vi "decodeObject.vi"(8 "error in (no error)":errorcluster, 10 "ByteArray":u8[](array[numeric])) -> (0 "error out":errorcluster, 1 "Variant":variant, 2 "RemainingBytes":u8[](array[numeric]), 3 "Type":string)   [LabVIEW 2016, in "MsgPack.lvlib"]
uses:
  MsgPack.lvlib
  <vilib>/Utility/error.llb/Error Cluster From Error Code.vi
  <vilib>/ErrorRing/Error Ring.xnode
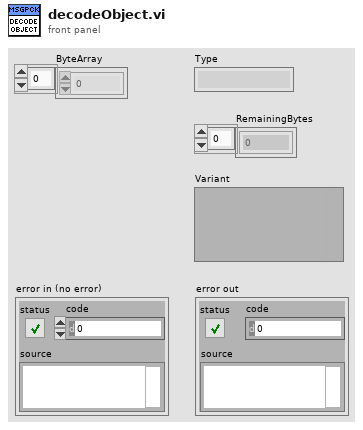
[diagram p1: front panel]
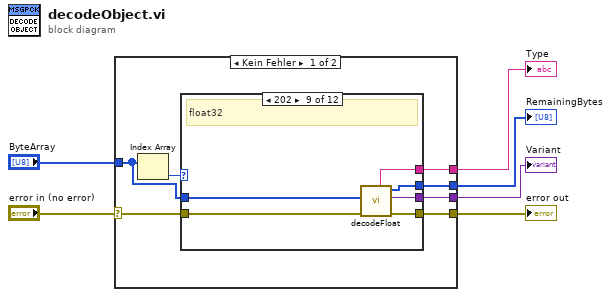
[diagram p0: block diagram]
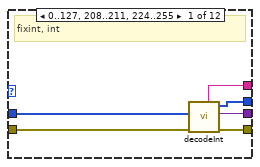
[diagram p2: hidden frame]
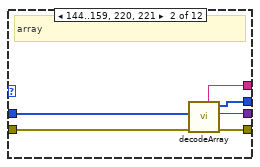
[diagram p3: hidden frame]
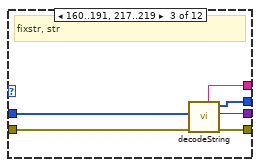
[diagram p4: hidden frame]
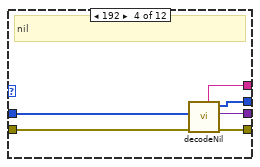
[diagram p5: hidden frame]
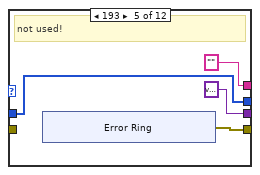
[diagram p6: hidden frame]
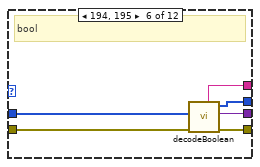
[diagram p7: hidden frame]
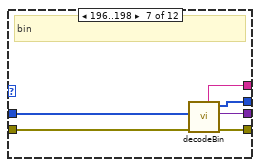
[diagram p8: hidden frame]
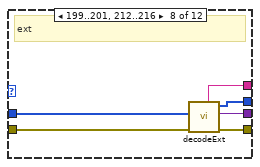
[diagram p9: hidden frame]
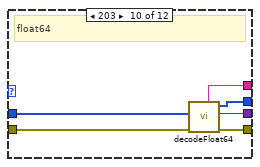
[diagram p10: hidden frame]
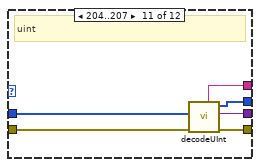
[diagram p11: hidden frame]
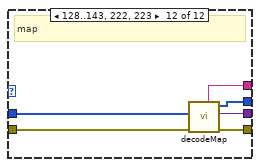
[diagram p12: hidden frame]
diagram:
  n1 = case shown="Kein Fehler" "error in (no error)" {
    selector: "error in (no error)" -> [w7 w90]
    tunnel: "ByteArray" -> [w12 w89]
    tunnel: [w11 _] -> w5
    tunnel: [w10 _] -> w4
    tunnel: [w9 w89] -> w3
    tunnel: [w8 w90] -> w2
    frame No Error {
      n2 = Index Array(array=w12) -> (element=w13:u8)  [unwired: 1 in]
      n3 = case shown="202" w13 {
        tunnel: w12 -> [w19 w24 w31 w34 w38 w52 w58 w64 w70 w76 w82 w88]
        tunnel: [w17 w22 w29 w37 w41 w50 w56 w62 w68 w74 w80 w84] -> w8
        tunnel: [w18 w21 w30 w36 variant ("variant") w51 w57 w63 w69 w75 w81 w86] -> w11
        tunnel: w7 -> [w16 w25 w26 w35 _ w49 w53 w59 w65 w71 w77 w87]
        tunnel: [w15 w23 w28 w33 w38 w47 w55 w61 w67 w72 w78 w85] -> w9
        tunnel: [w14 w20 w27 w32 "" ("Type") w48 w54 w60 w66 w73 w79 w83] -> w10
        frame 0..127, 208..211, 224..255 {
          # "fixint, int"
          n4 = call "decodeInt.vi"("error in (no error)"=w16, "ByteArray"=w19) -> ("error out"=w17:errorcluster, "variant"=w18:variant, "RemainingBytes"=w15:u8[], "Type"=w14:string)  [unwired: 5 in, 1 out]
        }
        frame 144..159, 220, 221 {
          # "array"
          n5 = call "decodeArray.vi"("error in (no error)"=w25, "ByteArray"=w24) -> ("error out"=w22:errorcluster, "variant"=w21:variant, "ByteArray"=w23:u8[], "Type"=w20:string)  [unwired: 6 in]
        }
        frame 160..191, 217..219 {
          # "fixstr, str"
          n6 = call "decodeString.vi"("error in (no error)"=w26, "ByteArray"=w31) -> ("error out"=w29:errorcluster, "variant"=w30:variant, "RemainingBytes"=w28:u8[], "Type"=w27:string)  [unwired: 5 in, 1 out]
        }
        frame 192 {
          # "nil"
          n7 = call "decodeNil.vi"("error in (no error)"=w35, "ByteArray"=w34) -> ("error out"=w37:errorcluster, "variant"=w36:variant, "RemainingBytes"=w33:u8[], "Type"=w32:string)  [unwired: 6 in]
        }
        frame 193 {
          # "not used!"
          n8 = xnode "Error Ring"() -> ("Fehler (Ausgang)"=w41:errorcluster)
        }
        frame 194, 195 {
          # "bool"
          n9 = call "decodeBoolean.vi"("error in (no error)"=w49, "ByteArray"=w52) -> ("error out"=w50:errorcluster, "variant"=w51:variant, "RemainingBytes"=w47:u8[], "Type"=w48:string)  [unwired: 5 in, 1 out]
        }
        frame 196..198 {
          # "bin"
          n10 = call "decodeBin.vi"("error in (no error)"=w53, "ByteArray"=w58) -> ("error out"=w56:errorcluster, "variant"=w57:variant, "RemainingBytes"=w55:u8[], "Type"=w54:string)  [unwired: 5 in, 1 out]
        }
        frame 199..201, 212..216 {
          # "ext"
          n11 = call "decodeExt.vi"("error in (no error)"=w59, "ByteArray"=w64) -> ("error out"=w62:errorcluster, "variant"=w63:variant, "RemainingBytes"=w61:u8[], "Type"=w60:string)  [unwired: 5 in, 1 out]
        }
        frame 202 {
          # "float32"
          n12 = call "decodeFloat.vi"("error in (no error)"=w65, "ByteArray"=w70) -> ("error out"=w68:errorcluster, "variant"=w69:variant, "RemainingBytes"=w67:u8[], "Type"=w66:string)  [unwired: 5 in, 1 out]
        }
        frame 203 {
          # "float64"
          n13 = call "decodeFloat64.vi"("error in (no error)"=w71, "ByteArray"=w76) -> ("error out"=w74:errorcluster, "variant"=w75:variant, "RemainingBytes"=w72:u8[], "Type"=w73:string)  [unwired: 5 in, 1 out]
        }
        frame 204..207 {
          # "uint"
          n14 = call "decodeUInt.vi"("error in (no error)"=w77, "ByteArray"=w82) -> ("error out"=w80:errorcluster, "variant"=w81:variant, "RemainingBytes"=w78:u8[], "Type"=w79:string)  [unwired: 5 in, 1 out]
        }
        frame 128..143, 222, 223 {
          # "map"
          n15 = call "decodeMap.vi"("error in (no error)"=w87, "ByteArray"=w88) -> ("error out"=w84:errorcluster, "variant"=w86:variant, "ByteArray"=w85:u8[], "Type"=w83:string)  [unwired: 6 in]
        }
      }
    }
    frame Error {
    }
  }
  "Variant" <- w5
  "Type" <- w4
  "RemainingBytes" <- w3
  "error out" <- w2
